vi "Update names group selector.vi"(8 "error in (no error)":errorcluster, 11 "Experiments_group in":refnum<class "Experiments_group.lvclass">) -> (0 "error out":errorcluster, 3 "Experiments_group out":refnum<class "Experiments_group.lvclass">)   [LabVIEW 2019, in "Experiments_group.lvclass"]
uses:
  Experiments_group.lvclass
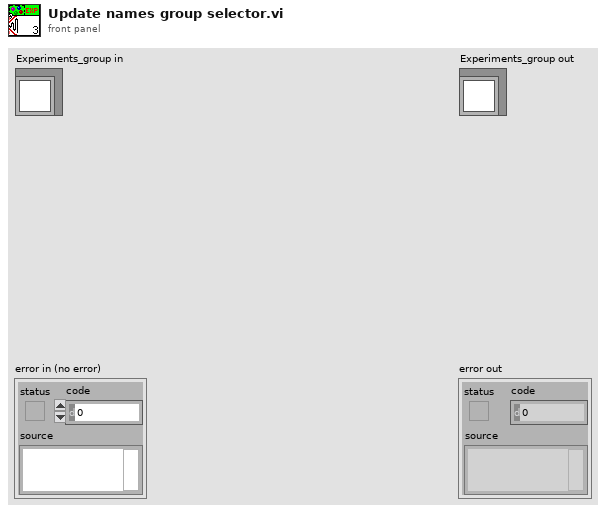
[diagram p1: front panel]
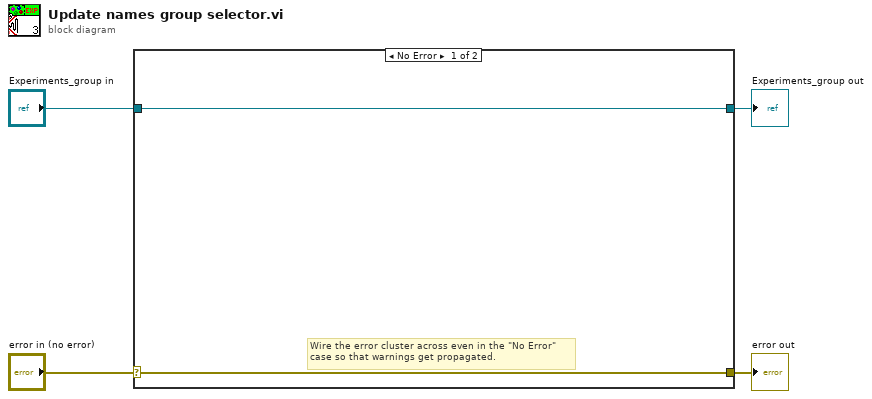
[diagram p0: block diagram]
diagram:
  n1 = case shown="No Error" "error in (no error)" {
    selector: "error in (no error)" -> [w5 w8]
    tunnel: [w5 w8] -> w3
    tunnel: [w6 w7] -> w1
    tunnel: "Experiments_group in" -> [w6 w7]
    frame No Error {
      # "Wire the error cluster across even in the \"No Error\"\ncase so that warnings get propagated."
    }
    frame Error {
    }
  }
  "error out" <- w3
  "Experiments_group out" <- w1
